vi "Factory.vi"(11 "Enum":T1) -> (3 "Caculator.lvlib:Strategy":refnum<class "Strategy.lvclass">)   [LabVIEW 2014, in "Caculator.lvlib"]
uses:
  Caculator.lvlib
  Enum.ctl
  Strategy_class/Strategy.lvclass
  Add_class/Add.lvclass
  Subtract_class/Subtract.lvclass
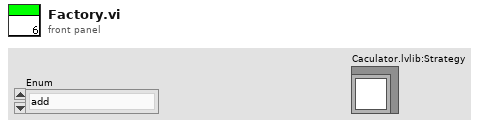
[diagram p1: front panel]
types:
  T1 = typedef "Caculator.lvlib/Enum.ctl" = enum16{"add", "subtract"}
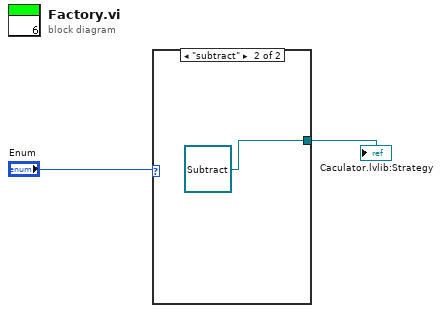
[diagram p0: block diagram]
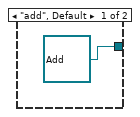
[diagram p2: hidden frame]
diagram:
  n1 = case shown="\"subtract\"" "Enum" {
    tunnel: [refnum<class "Add.lvclass"> refnum ("Caculator.lvlib:Add") refnum<class "Subtract.lvclass"> refnum ("Caculator.lvlib:Subtract")] -> w1
    frame "add", Default {
    }
    frame "subtract" {
    }
  }
  "Caculator.lvlib:Strategy" <- w1
